vi "GetSectionMap.vi"(8 "error in (no error)":errorcluster caption="에러 입력(에러 없음)", 10 "Section":T2(ring)=enum."DataSection", 11 "ABFFIO 입력":refnum<class "ABFFIO.lvclass">) -> (0 "error out":errorcluster caption="에러 출력", 2 "SectionMap":T1, 3 "ABFFIO 출력":refnum<class "ABFFIO.lvclass">)   [LabVIEW 2017, in "ABFFIO.lvclass"]
uses:
  ABFFIO.lvclass
  ABFFIO.lvclass/ABFFIO.ctl
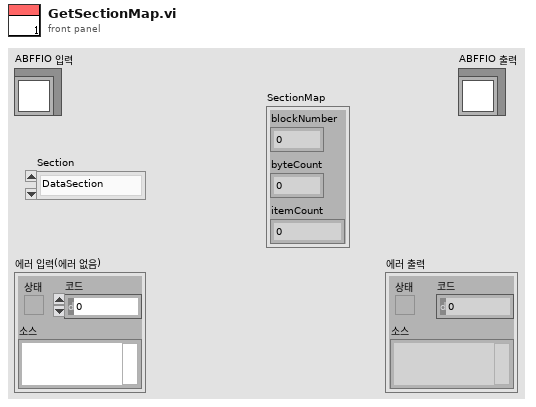
[diagram p1: front panel]
types:
  T1 = cluster{"blockNumber":u32, "byteCount":u32, "itemCount":u32}
  T2 = enum16{"ProtocolSection", "ADCSection", "DACSection", "EpochSection", "ADCPerDACSection", "EpochPerDACSection", "StringsSection", "DataSection", "TagSection"}
  T3 = enum16{"big-endian, network order", "native, host order", "little-endian"}
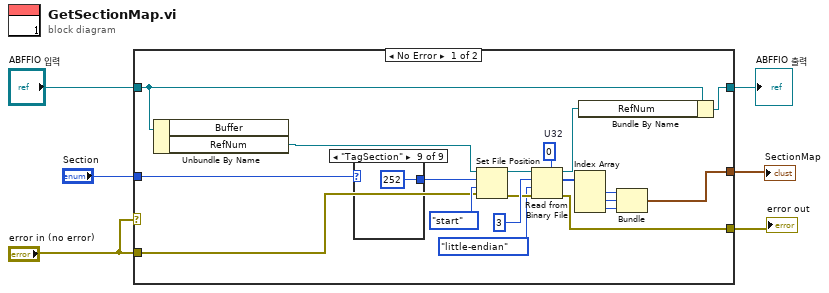
[diagram p0: block diagram]
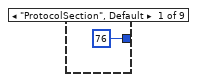
[diagram p2: hidden frame]
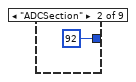
[diagram p3: hidden frame]
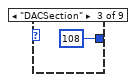
[diagram p4: hidden frame]
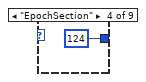
[diagram p5: hidden frame]
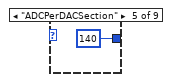
[diagram p6: hidden frame]
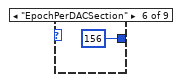
[diagram p7: hidden frame]
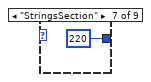
[diagram p8: hidden frame]
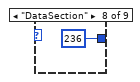
[diagram p9: hidden frame]
diagram:
  n1 = case shown="No Error" "error in (no error)" {
    selector: "error in (no error)" -> [_ w36]
    tunnel: [w11 w36] -> w6
    tunnel: [w7 w35] -> w4
    tunnel: "ABFFIO 입력" -> [w8 w35]
    tunnel: "Section" -> [w25 _]
    tunnel: [w24 _] -> w2
    tunnel: "error in (no error)" -> [w10 _]
    frame No Error {
      w16 = u32 0  # U32
      n2 = Unbundle By Name(w8) -> ("RefNum"=w17:refnum<file>)  [unwired: 1 out]
      n3 = case shown="\"TagSection\"" w25 {
        tunnel: [76 92 ("오프셋(0)") 108 124 140 156 220 236 252] -> w22
        frame "ProtocolSection", Default {
        }
        frame "ADCSection" {
        }
        frame "DACSection" {
        }
        frame "EpochSection" {
        }
        frame "ADCPerDACSection" {
        }
        frame "EpochPerDACSection" {
        }
        frame "StringsSection" {
        }
        frame "DataSection" {
        }
        frame "TagSection" {
        }
      }
      n4 = Set File Position(offset (in bytes) (0)=w22, refnum=w17, from (0:start)=enum16{"start", "end", "current"}."start", error in=w10) -> (refnum out=w19:refnum<file>, error out=w20:errorcluster)
      n5 = Read from Binary File(5:w16, 8:w20, 9:T3."little-endian" ("byte order (0:big-endian, network order)"), 10:3 ("count (1)"), 11:w19) -> (0:w11:errorcluster, 2:w15:u32[], 3:w9:refnum<file>)  [unwired: 1 in, 1 out]
      n6 = Index Array(array=w15) -> (element #1=w14:u32, element #2=w13:u32, element #3=w12:u32)  [unwired: 3 in]
      n7 = Bundle By Name(cluster=w8, "RefNum"=w9) -> (w7:refnum<class "ABFFIO.lvclass">)
      n8 = Bundle("U32"=w14, "U32"=w13, "U32"=w12) -> (w24:cluster{"U32":u32, "U32":u32, "U32":u32})  [unwired: 1 in]
    }
    frame Error {
    }
  }
  "error out" <- w6
  "ABFFIO 출력" <- w4
  "SectionMap" <- w2
